vi "Configure Comparator.vi"(0 "VISA resource name":refnum<visa-resource-name>, 1 "Total Number of Bins (0)":i32=1 min=1 max=9 step=1, 5 "COMP Status (T: Enable)":bool=TRUE, 7 "Limit Mode (0: ABS)":i32(ring) items=["ABS", "PER", "SEQ"], 9 "AUX Status (F: Disable)":bool, 11 "error in (no error)":errorcluster, 12 "Beep Mode (0: OFF)":i32(ring) items=["OFF", "PASS", "FAIL"]) -> (4 "VISA resource name out":refnum<visa-resource-name>, 15 "error out":errorcluster)   [LabVIEW 2014, in "LCR Meter.lvlib"]
doc: "Sets the Comparator Parameter."
uses:
  <instrlib>/LCR Meter/Examples/LCR Meter Acquire Single_1 Folder/LCR Meter.lvlib
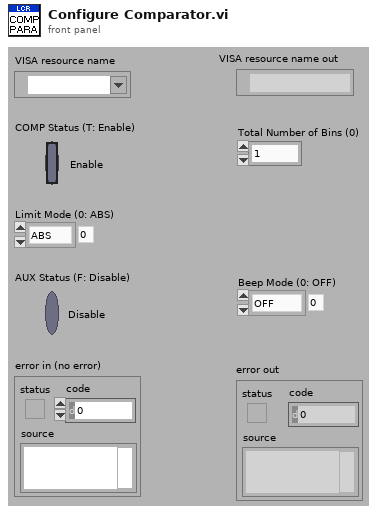
[diagram p1: front panel]
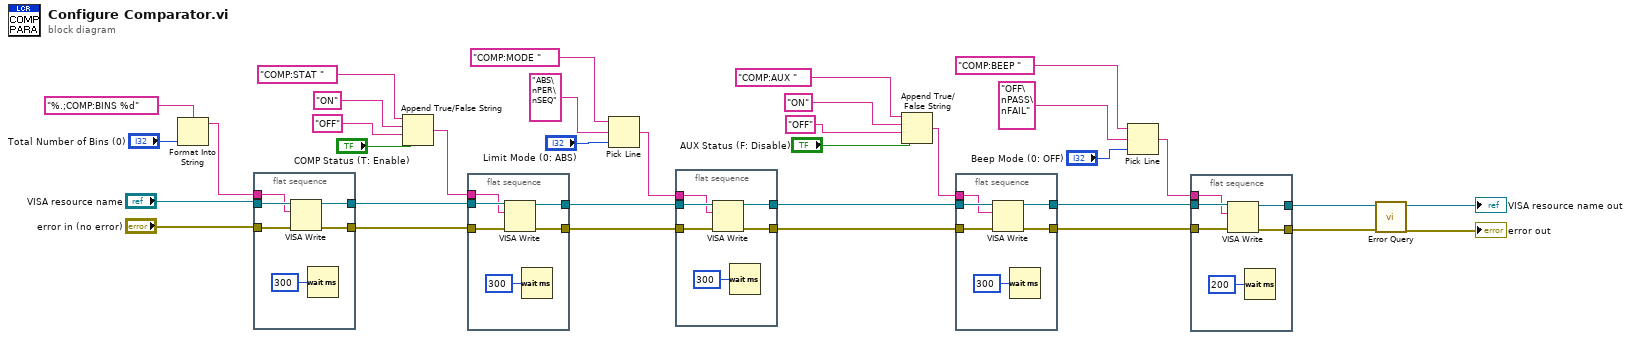
[diagram p0: block diagram]
diagram:
  n1 = Format Into String(format string="%.;COMP:BINS %d", "Total Number of Bins (0)") -> (resulting string=w5:string)  [unwired: 2 in, 1 out]
  n2 = flat-sequence {
    tunnel: "VISA resource name" -> [w40]
    tunnel: "error in (no error)" -> [w39]
    tunnel: [w38] -> w7
    tunnel: [w37] -> w6
    tunnel: w5 -> [w36]
    frame #0 {
      n3 = VISA Write(VISA resource name=w40, write buffer=w36, error in (no error)=w39) -> (VISA resource name out=w38:refnum<visa-resource-name>, error out=w37:errorcluster)  [unwired: 1 out]
      n4 = Wait (ms)(milliseconds to wait=u32 300) -> ()  [unwired: 1 out]
    }
  }
  n5 = Append True/False String(1:"COMP Status (T: Enable)", 2:"OFF", 3:"ON", 4:"COMP:STAT " ("string (\"\")")) -> (0:w17:string)
  n6 = flat-sequence {
    tunnel: w7 -> [w46]
    tunnel: w6 -> [w45]
    tunnel: [w44] -> w24
    tunnel: [w43] -> w23
    tunnel: w17 -> [w42]
    frame #0 {
      n7 = VISA Write(VISA resource name=w46, write buffer=w42, error in (no error)=w45) -> (VISA resource name out=w44:refnum<visa-resource-name>, error out=w43:errorcluster)  [unwired: 1 out]
      n8 = Wait (ms)(milliseconds to wait=u32 300) -> ()  [unwired: 1 out]
    }
  }
  n9 = Pick Line(string ("")="COMP:MODE ", multi-line string="ABS\nPER\nSEQ", line index="Limit Mode (0: ABS)") -> (output string=w18:string)
  n10 = flat-sequence {
    tunnel: w24 -> [w52]
    tunnel: w23 -> [w51]
    tunnel: [w50] -> w22
    tunnel: [w49] -> w21
    tunnel: w18 -> [w48]
    frame #0 {
      n11 = VISA Write(VISA resource name=w52, write buffer=w48, error in (no error)=w51) -> (VISA resource name out=w50:refnum<visa-resource-name>, error out=w49:errorcluster)  [unwired: 1 out]
      n12 = Wait (ms)(milliseconds to wait=u32 300) -> ()  [unwired: 1 out]
    }
  }
  n13 = Append True/False String(1:"AUX Status (F: Disable)", 2:"OFF", 3:"ON", 4:"COMP:AUX " ("string (\"\")")) -> (0:w19:string)
  n14 = flat-sequence {
    tunnel: w22 -> [w58]
    tunnel: w21 -> [w57]
    tunnel: [w56] -> w4
    tunnel: [w55] -> w3
    tunnel: w19 -> [w54]
    frame #0 {
      n15 = VISA Write(VISA resource name=w58, write buffer=w54, error in (no error)=w57) -> (VISA resource name out=w56:refnum<visa-resource-name>, error out=w55:errorcluster)  [unwired: 1 out]
      n16 = Wait (ms)(milliseconds to wait=u32 300) -> ()  [unwired: 1 out]
    }
  }
  n17 = Pick Line(string ("")="COMP:BEEP ", multi-line string="OFF\nPASS\nFAIL", line index="Beep Mode (0: OFF)") -> (output string=w20:string)
  n18 = flat-sequence {
    tunnel: w4 -> [w64]
    tunnel: w3 -> [w63]
    tunnel: [w62] -> w2
    tunnel: [w61] -> w1
    tunnel: w20 -> [w60]
    frame #0 {
      n19 = VISA Write(VISA resource name=w64, write buffer=w60, error in (no error)=w63) -> (VISA resource name out=w62:refnum<visa-resource-name>, error out=w61:errorcluster)  [unwired: 1 out]
      n20 = Wait (ms)(milliseconds to wait=u32 200) -> ()  [unwired: 1 out]
    }
  }
  n21 = call <instrlib>:"Error Query.vi"("error in (no error)"=w1, "VISA resource name"=w2) -> ("error out"=→"error out":errorcluster, "VISA resource name out"=→"VISA resource name out":refnum<visa-resource-name>)  [unwired: 6 in, 2 out]
